vi "End Group.vi"(8 "Error In":errorcluster, 11 "Group Item References":refnum<vi>[](array[refnum])) -> (0 "Error Out":errorcluster)   [LabVIEW 2019, in "LSS.lvlib"]
doc: "Use this VI to clear a grouping of control. The tag used to identify controls as a group is reset to an empty string when this VI is run.\n\n<b>Inputs:</b>\n<b>Group Item References</b> - Array of references to objects that will be removed from all groups. This can end one group, or all groups at once.\n<b>Error In</b> - Standard Error in terminal\n\n<b>Outputs:</b>\n<b>Error Out</b> - Standard Error out terminal"
uses:
  LSS.lvlib
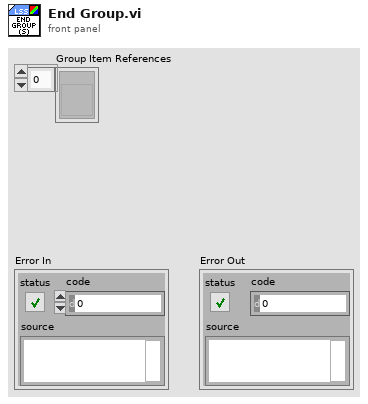
[diagram p1: front panel]
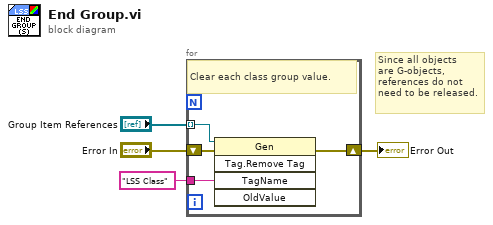
[diagram p0: block diagram]
diagram:
  # "Since all objects\nare G-objects,\nreferences do not\nneed to be released."
  n1 = for {
    tunnel: "LSS Class" ("Tag Name") -> [w8]
    tunnel: "Group Item References" -> [w6] mode=indexing
    shift-right: [w7] -> w2
    shift-left: "Error In" -> [w5]
    # "Clear each class group value."
    n2 = invoke class="Gen" method="Tag.Remove Tag"(reference=w6, error in=w5, "TagName"=w8) -> (error out=w7:errorcluster)  [unwired: 2 in, 4 out]
  }
  "Error Out" <- w2
